vi "parse comma separated string.vi"(11 "String":string) -> (3 "Array":string[](array[string]))   [LabVIEW 2015, in "SLSC Switch.lvclass"]
uses:
  SLSC Switch.lvclass
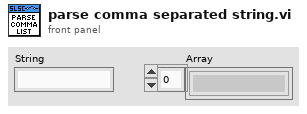
[diagram p1: front panel]
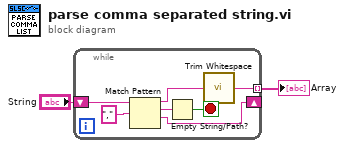
[diagram p0: block diagram]
diagram:
  n1 = while {
    shift-right: [w9] -> _
    shift-left: "String" -> [w8]
    tunnel: [w3] -> w1 mode=indexing
    stop <- w6 stop-if-true
    n2 = Match Pattern(string=w8, regular expression="," ("search string/char (-)")) -> (before substring=w4:string, match substring=w5:string, after substring=w9:string)  [unwired: 1 in, 1 out]
    n3 = Empty String/Path?(string/path=w5) -> (empty?=w6:bool)
    n4 = call <vilib>:"Trim Whitespace.vi"("string"=w4) -> ("trimmed string"=w3:string)  [unwired: 1 in]
  }
  "Array" <- w1
